vi "Log_ADAM_scan_table.vi"() -> ()   [LabVIEW 2013]
uses:
  ADAM Client/Sub VIs/ADAM Controls/Channel_State.ctl
  Anemometry/Anemometry Sub Vis/Globals/Constants_global.vi
  Anemometry/Anemometry Sub Vis/Globals/Preference_global.vi
  ADAM_Global.vi
  Anemometry/Anemometry Sub Vis/Globals/Meas_global.vi
panel:
  in  "Ventilate Lab if temp above":dbl=21.5
  in  "Averaging time (Seconds)":dbl=60.0
  out "Current time":string
  out "Started Time":string
  in  "stop":bool
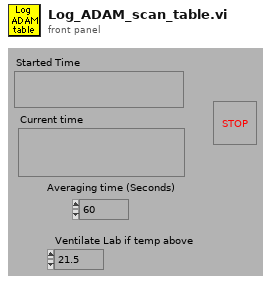
[diagram p1: front panel]
types:
  T1 = enum16{"On", "Off", "Always On", "Always Off", "Delete"}
  T2 = typedef "Channel_State.ctl" = enum16{"On", "Off", "Always On", "Always Off"}
  T3 = enum16{"Load ADAM setup from excel file", "Save ADAM setup to excel file"}
  T4 = cluster{"second":i32, "minute":i32, "hour":i32, "day of month":i32, "month":i32, "year":i32, "day of week":i32, "day of year":i32, "is DST":i32}
  T5 = typedef "Client_State_Cluster.ctl" = cluster{"Client Name":string, "Traverse level State":T6, "People to Email":string[], "Next Contact Time":dbl}
  T6 = typedef "Traverse_Level_State.ctl" = enum16{"Running", "Complete"}
  T7 = typedef "Server_Control.ctl" = cluster{"Channel Name to control":string, "Channel sharing":enum16{"Channel Unshared", "Channel Shared by Rig", "Channel Shared by Group"}, "Default Value":dbl, "Client Array":string[], "Time Stamp":timestamp, "Do Not Reset":bool}
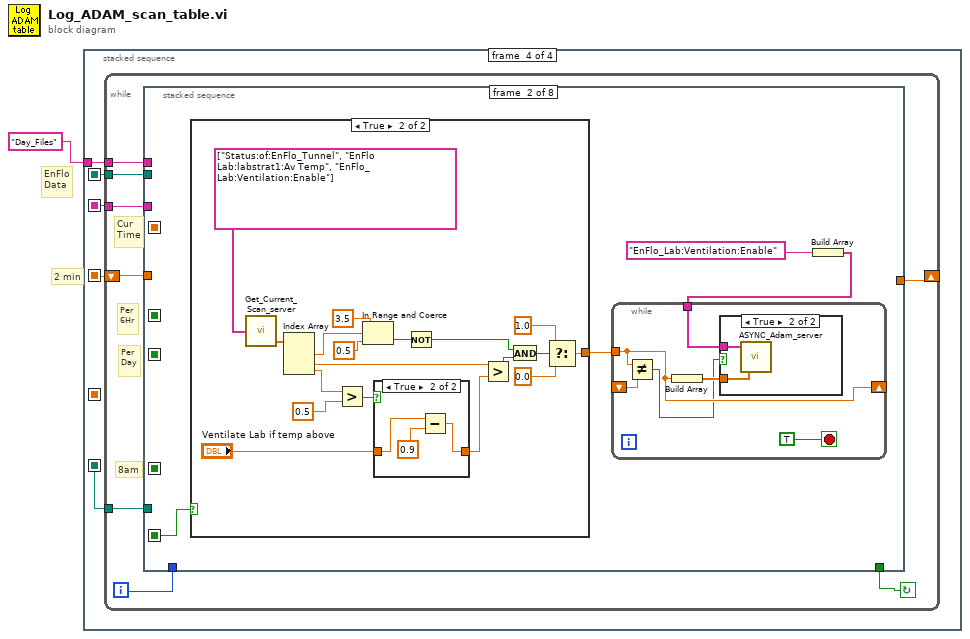
[diagram p0: block diagram]
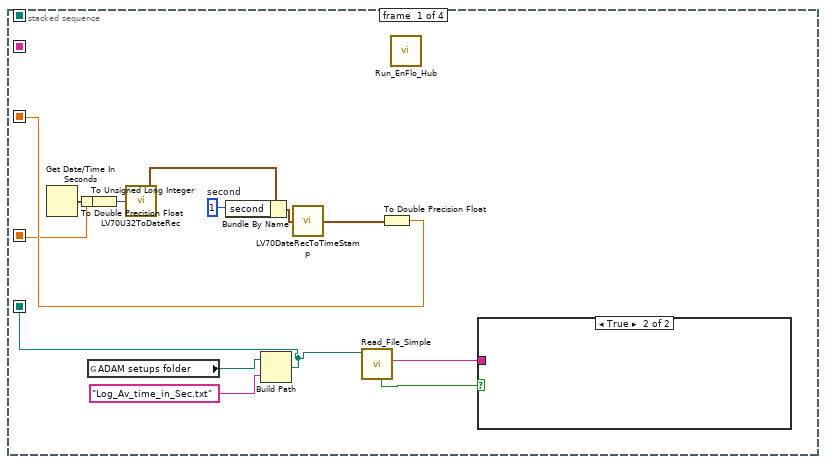
[diagram p2: hidden frame]
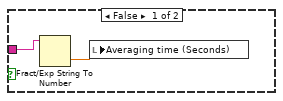
[diagram p3: hidden frame]
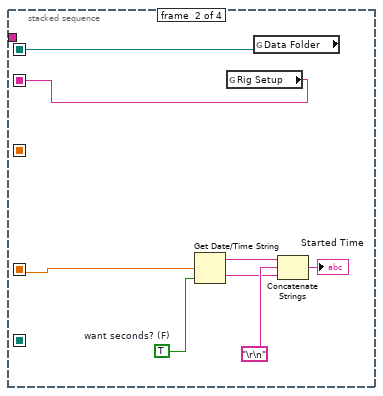
[diagram p4: hidden frame]
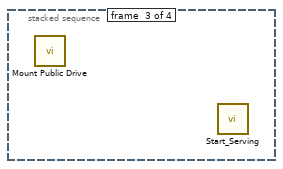
[diagram p5: hidden frame]
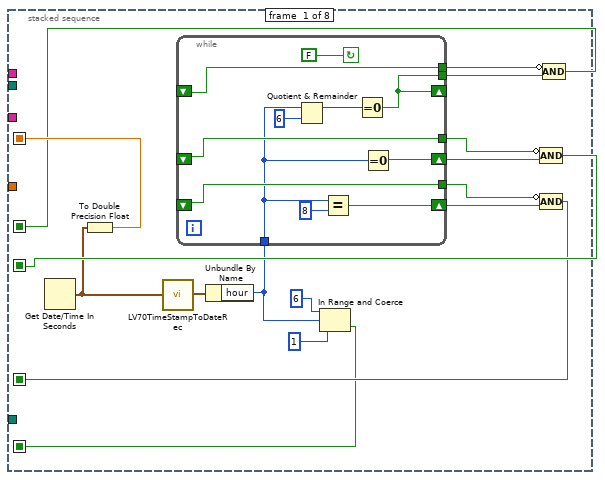
[diagram p6: hidden frame]
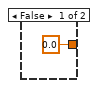
[diagram p8: hidden frame]
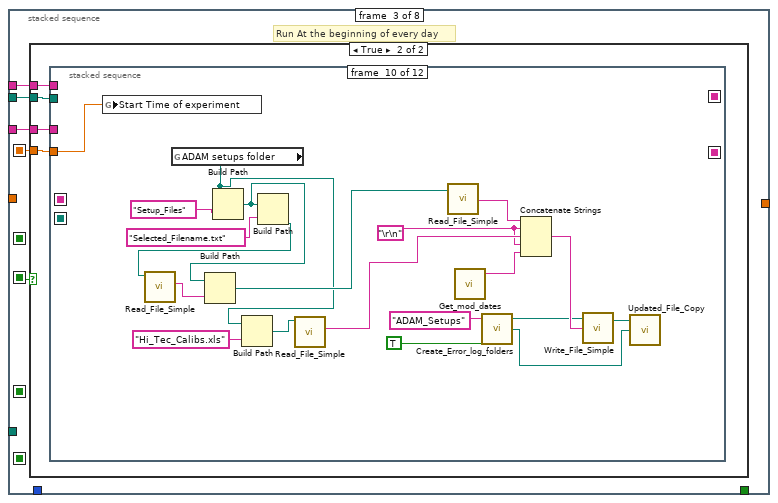
[diagram p10: hidden frame]
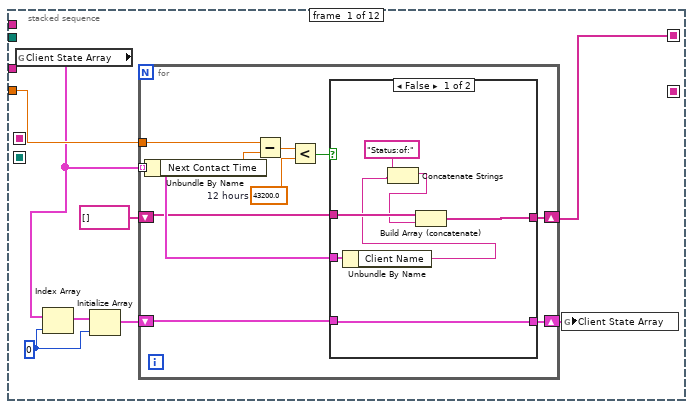
[diagram p12: hidden frame]
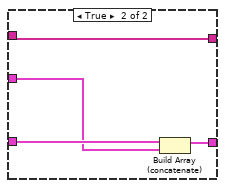
[diagram p13: hidden frame]
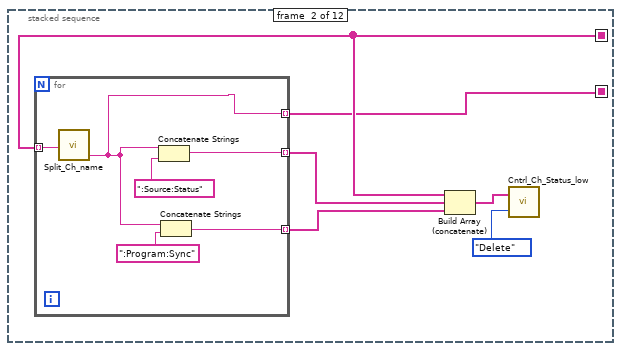
[diagram p14: hidden frame]
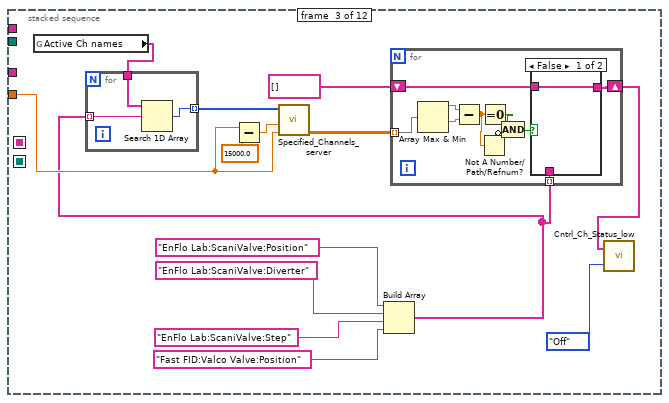
[diagram p15: hidden frame]
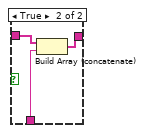
[diagram p16: hidden frame]
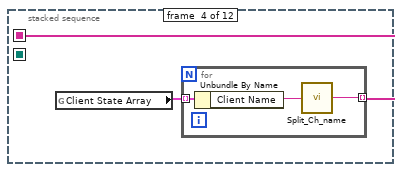
[diagram p17: hidden frame]
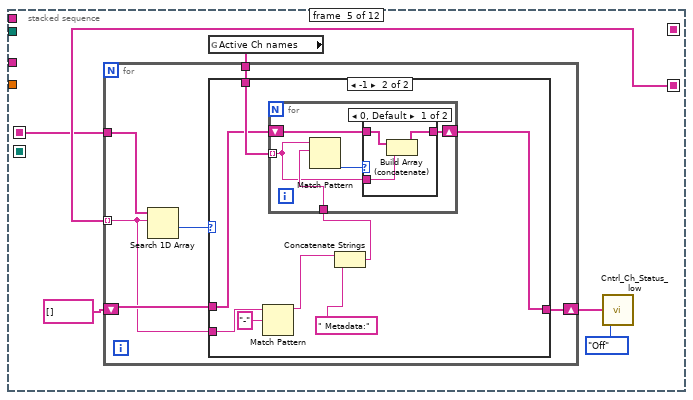
[diagram p18: hidden frame]
diagram:
  # "EnFlo\nData"
  # "2 min"
  n1 = stacked-sequence {
    seq-local: [w12 _ _ _] -> [_ _ _ w29]
    seq-local: [w11 _ _ _] -> [_ w24 _ _]
    seq-local: [_ w18 _ _] -> [_ _ _ w28]
    seq-local: [w4 _ _ _] -> [_ _ _ w26]
    seq-local: [_ w17 _ _] -> [_ _ _ w25]
    tunnel: "Day_Files" ("Input Element") -> [_ _ _ w27]
    frame #0 {
      w14 = 1  # second
      n2 = Get Date/Time In Seconds() -> (seconds since 1Jan1904=w8:timestamp)
      n3 = To Double Precision Float(number=w8) -> (double precision float=w11:dbl)
      n4 = global read "Constants_global.vi" "ADAM setups folder"() -> (w6:path)
      n5 = To Unsigned Long Integer(number=w11) -> (unsigned 32bit integer=w10:u32)
      n6 = call <vilib>:"LV70U32ToDateRec.vi"("Time"=w10) -> ("date time rec"=w9:T4)
      n7 = Bundle By Name(cluster=w9, "second"=w14) -> (w13:T4)
      n8 = Build Path(base path=w6, name or relative path="Log_Av_time_in_Sec.txt") -> (appended path=w4:path)
      n9 = call <vilib>:"LV70DateRecToTimeStamp.vi"("date time rec"=w13) -> ("Time Stamp"=w7:timestamp)
      n10 = call "Read_File_Simple.vi"("Filename"=w4) -> ("Error?"=w2:bool, "string"=w3:string)  [unwired: 2 in, 6 out]
      n11 = To Double Precision Float(number=w7) -> (double precision float=w12:dbl)
      n12 = call "Run_EnFlo_Hub.vi"() -> ()  [unwired: 8 out]
      n13 = case shown="True" w2 {
        tunnel: w3 -> [w16 _]
        frame False {
          n14 = Fract/Exp String To Number(string=w16) -> (number=w15:dbl)  [unwired: 4 out]
          n15 = local write "Averaging time (Seconds)"(w15) -> ()
        }
        frame True {
        }
      }
    }
    frame #1 {
      w23 = TRUE  # want seconds? (F)
      n16 = Get Date/Time String(seconds (now)=w24, want seconds? (F)=w23) -> (date string=w21:string, time string=w20:string)  [unwired: 1 out]
      n17 = global read "Preference_global.vi" "Rig Setup"() -> (w17:string)
      n18 = global read "Constants_global.vi" "Data Folder"() -> (w18:path)
      n19 = Concatenate Strings(w21, "\r\n", w20) -> (→"Started Time":string)
    }
    frame #2 {
      n20 = call "Mount Public Drive.vi"() -> ()  [unwired: 12 in]
      n21 = call "Start_Serving.vi"() -> ()  [unwired: 1 out]
    }
    frame #3 {
      n22 = while {
        tunnel: w28 -> [w35]
        shift-left: w29 -> [w37]
        shift-right: [w36] -> _
        tunnel: w27 -> [w32]
        tunnel: w26 -> [w31]
        tunnel: w25 -> [w30]
        i -> [w34]
        stop <- w33 continue-if-true
        # "8am"
        # "Per\n6Hr"
        # "Per\nDay"
        # "Cur\nTime"
        n23 = stacked-sequence {
          seq-local: [w46 _ _ _ _ _ _ _] -> [_ _ w104 _ _ _ _ _]
          seq-local: [w52 _ _ _ _ _ _ _] -> [_ _ w103 w330 w349 _ _ _]
          seq-local: [w49 _ _ _ _ _ _ _] -> [_ _ _ _ _ _ _ _]
          seq-local: [w42 _ _ _ _ _ _ _] -> [_ _ _ w326 _ _ _ _]
          seq-local: [w38 _ _ _ _ _ _ _] -> [_ w68 _ _ _ _ _ _]
          tunnel: [_ _ _ _ _ w351 _ _] -> w36
          tunnel: w37 -> [_ _ _ _ _ w352 _ _]
          tunnel: w35 -> [_ _ w102 w329 _ w359 _ _]
          tunnel: w34 -> [_ _ _ _ _ _ _ _]
          tunnel: [_ _ _ _ _ _ _ w391] -> w33
          tunnel: w32 -> [_ _ w101 w328 _ w360 _ _]
          tunnel: w31 -> [_ _ _ _ _ _ _ w390]
          tunnel: w30 -> [_ _ w100 w327 _ w353 _ _]
          frame #0 {
            n24 = Get Date/Time In Seconds() -> (seconds since 1Jan1904=w45:timestamp)
            n25 = To Double Precision Float(number=w45) -> (double precision float=w52:dbl)
            n26 = call <vilib>:"LV70TimeStampToDateRec.vi"("time stamp"=w45) -> ("date time rec"=w53:T4)
            n27 = Unbundle By Name(w53) -> ("hour"=w41:i32)
            n28 = while {
              tunnel: [w59] -> w47
              shift-left: _ -> [w59]
              shift-right: [w60] -> w48
              tunnel: [w61] -> w50
              tunnel: [w62] -> w51
              tunnel: w41 -> [w56]
              shift-left: _ -> [w61]
              shift-right: [w62] -> _
              tunnel: [w57] -> w44
              shift-right: [w54] -> w43
              shift-left: _ -> [w57]
              stop <- FALSE continue-if-true
              n29 = Quotient & Remainder(x=w56, y=6) -> (x-y*floor(x/y)=w63:i32)  [unwired: 1 out]
              n30 = Equal?(x=w56, y=8) -> (x = y?=w54:bool)
              n31 = Equal To 0?(x=w63) -> (x = 0?=w62:bool)
              n32 = Equal To 0?(x=w56) -> (x = 0?=w60:bool)
            }
            n33 = In Range and Coerce(upper limit=6, x=w41, lower limit=1) -> (In Range?=w38:bool)  [unwired: 1 out]
            n34 = Compound Arithmetic op=AND(invert w47, w48) -> (w46:bool)
            n35 = Compound Arithmetic op=AND(invert w44, w43) -> (w42:bool)
            n36 = Compound Arithmetic op=AND(invert w50, w51) -> (w49:bool)
          }
          frame #1 {
            n37 = case shown="True" w68 {
              tunnel: [0.0 ("f") w88] -> w65
              frame False {
              }
              frame True {
                n38 = call "Get_Current_Scan_server.vi"("Desired Channels"=string[] ["Status:of:EnFlo_Tunnel", "EnFlo Lab:labstrat1:Av Temp", "EnFlo_Lab:Ventilation:Enable"]) -> ("Numerical Values"=w94:dbl[])  [unwired: 2 out]
                n39 = Index Array(array=w94) -> (element #1=w87:dbl, element #2=w93:dbl, element #3=w82:dbl)  [unwired: 3 in]
                n40 = Greater?(x=w82, y=0.5) -> (0:w80:bool)
                n41 = In Range and Coerce(upper limit=3.5, x=w87, lower limit=0.5) -> (In Range?=w84:bool)  [unwired: 1 out]
                n42 = case shown="True" w80 {
                  tunnel: [w96 w97] -> w79
                  tunnel: "Ventilate Lab if temp above" -> [w96 w99]
                  frame False {
                  }
                  frame True {
                    n43 = Subtract(x=w99, y=0.9) -> (x-y=w97:dbl)
                  }
                }
                n44 = Not(x=w84) -> (.not. x?=w83:bool)
                n45 = Greater?(x=w93, y=w79) -> (0:w92:bool)
                n46 = And(x=w83, y=w92) -> (x .and. y?=w91:bool)
                n47 = Select(t=1.0, s=w91, f=0.0) -> (s? t:f=w88:dbl)
              }
            }
            n48 = Build Array("EnFlo_Lab:Ventilation:Enable") -> (w66:string[])
            n49 = while {
              shift-right: [w72] -> _
              shift-left: _ -> [w73]
              tunnel: w65 -> [w72]
              tunnel: w66 -> [w70]
              stop <- TRUE stop-if-true
              n50 = Not Equal?(x=w72, y=w73) -> (x != y?=w69:bool)
              n51 = Build Array(w72) -> (w74:dbl[])
              n52 = case shown="True" w69 {
                tunnel: w74 -> [_ w76]
                tunnel: w70 -> [_ w75]
                frame False {
                }
                frame True {
                  n53 = call "ASYNC_Adam_server.vi"("Values"=w76, "Channel Names"=w75) -> ()  [unwired: 1 in, 3 out]
                }
              }
            }
          }
          frame #2 {
            # "Run At the beginning of every day"
            n54 = case shown="True" w104 {
              tunnel: w103 -> [_ w108]
              tunnel: w102 -> [_ w107]
              tunnel: w101 -> [_ w106]
              tunnel: w100 -> [_ w105]
              frame False {
              }
              frame True {
                n55 = stacked-sequence {
                  seq-local: [w109 _ _ _ _ _ _ _ _ _ _ _] -> [_ w143 _ _ _ _ _ _ w263 _ _ _]
                  seq-local: [_ w139 _ _ _ _ _ _ _ _ _ _] -> [_ _ _ _ w191 _ _ _ _ _ _ _]
                  seq-local: [_ _ _ w181 _ _ _ _ _ _ _ _] -> [_ _ _ _ w188 _ _ _ _ _ _ _]
                  seq-local: [_ _ _ _ _ _ _ _ _ _ w312 _] -> [_ _ _ _ _ _ _ _ _ _ _ w316]
                  tunnel: w108 -> [w116 _ w160 _ _ _ _ _ _ w310 _ w317]
                  tunnel: w107 -> [_ _ _ _ _ _ _ _ _ _ _ _]
                  tunnel: w106 -> [_ _ _ _ _ _ _ _ _ _ _ _]
                  tunnel: w105 -> [_ _ _ _ _ _ _ _ _ _ _ _]
                  frame #0 {
                    w114 = 0 ("Index")
                    n56 = global read "ADAM_Global.vi" "Client State Array"() -> (w115:T5[])
                    n57 = Index Array(array=w115, index=w114) -> (element=w113:T5)
                    n58 = Initialize Array(w113, w114) -> (w112:T5[])
                    n59 = for {
                      tunnel: w115 -> [w119] mode=indexing
                      shift-right: [w120] -> w111
                      shift-left: w112 -> [w121]
                      tunnel: w116 -> [w126]
                      shift-right: [w117] -> w109
                      shift-left: string[] [] -> [w118]
                      w123 = 43200.0  # 12 hours
                      n60 = Unbundle By Name(w119) -> ("Next Contact Time"=w125:dbl)
                      n61 = Subtract(x=w126, y=w125) -> (x-y=w124:dbl)
                      n62 = Less?(x=w124, y=w123) -> (x < y?=w122:bool)
                      n63 = case shown="False" w122 {
                        tunnel: w121 -> [w133 w137]
                        tunnel: [w133 w136] -> w120
                        tunnel: w119 -> [w132 w135]
                        tunnel: w118 -> [w131 w134]
                        tunnel: [w130 w134] -> w117
                        frame False {
                          n64 = Unbundle By Name(w132) -> ("Client Name"=w128:string)
                          n65 = Concatenate Strings("Status:of:", w128) -> (w127:string)
                          n66 = Build Array (concatenate)(w131, w127) -> (w130:string[])
                        }
                        frame True {
                          n67 = Build Array (concatenate)(w137, w135) -> (w136:T5[])
                        }
                      }
                    }
                    n68 = global write "ADAM_Global.vi" "Client State Array"(w111) -> ()
                  }
                  frame #1 {
                    n69 = for {
                      tunnel: w143 -> [w149] mode=indexing
                      tunnel: [w146] -> w141 mode=indexing
                      tunnel: [w145] -> w140 mode=indexing
                      tunnel: [w144] -> w139 mode=indexing
                      n70 = call "Split_Ch_name.vi"("Ch name"=w149) -> ("Low level"=w144:string)  [unwired: 2 out]
                      n71 = Concatenate Strings(w144, ":Source:Status") -> (w146:string)
                      n72 = Concatenate Strings(w144, ":Program:Sync") -> (w145:string)
                    }
                    n73 = Build Array (concatenate)(w143, w141, w140) -> (w142:string[])
                    n74 = call "Cntrl_Ch_Status_low.vi"("Mode"=T1."Delete", "Channel names"=w142) -> ()  [unwired: 1 out]
                  }
                  frame #2 {
                    n75 = global read "ADAM_Global.vi" "Active Ch names"() -> (w163:string[])
                    n76 = Subtract(x=w160, y=15000.0) -> (x-y=w158:dbl)
                    n77 = Build Array("EnFlo Lab:ScaniValve:Position", "EnFlo Lab:ScaniValve:Diverter", "EnFlo Lab:ScaniValve:Step", "Fast FID:Valco Valve:Position") -> (w156:string[])
                    n78 = for {
                      tunnel: w163 -> [w180]
                      tunnel: w156 -> [w179] mode=indexing
                      tunnel: [w178] -> w161 mode=indexing
                      n79 = Search 1D Array(1D array=w180, element=w179) -> (index of element=w178:i32)  [unwired: 1 out]
                    }
                    n80 = call "Specified_Channels_server.vi"("End time"=w160, "Start time"=w158, "Requested channels"=w161) -> ("Output array"=w157:dbl[][])  [unwired: 2 in, 4 out]
                    n81 = for {
                      tunnel: w157 -> [w170] mode=indexing
                      shift-right: [w171] -> w151
                      shift-left: string[] [] -> [w165]
                      tunnel: w156 -> [w166] mode=indexing
                      n82 = Array Max & Min(array=w170) -> (max value=w173:dbl, min value=w172:dbl)  [unwired: 2 out]
                      n83 = Subtract(x=w173, y=w172) -> (x-y=w169:dbl)
                      n84 = Not A Number/Path/Refnum?(number/path/refnum=w169) -> (NaN/Path/Refnum?=w167:bool)
                      n85 = Equal To 0?(x=w169) -> (x = 0?=w164:bool)
                      n86 = Compound Arithmetic op=AND(w164, invert w167) -> (w168:bool)
                      n87 = case shown="False" w168 {
                        tunnel: [w174 w177] -> w171
                        tunnel: w166 -> [_ w176]
                        tunnel: w165 -> [w174 w175]
                        frame False {
                        }
                        frame True {
                          n88 = Build Array (concatenate)(w175, w176) -> (w177:string[])
                        }
                      }
                    }
                    n89 = call "Cntrl_Ch_Status_low.vi"("Mode"=T1."Off", "Channel names"=w151) -> ()  [unwired: 1 out]
                  }
                  frame #3 {
                    n90 = global read "ADAM_Global.vi" "Client State Array"() -> (w182:T5[])
                    n91 = for {
                      tunnel: w182 -> [w185] mode=indexing
                      tunnel: [w183] -> w181 mode=indexing
                      n92 = Unbundle By Name(w185) -> ("Client Name"=w184:string)
                      n93 = call "Split_Ch_name.vi"("Ch name"=w184) -> ("Middle"=w183:string)  [unwired: 2 out]
                    }
                  }
                  frame #4 {
                    n94 = global read "ADAM_Global.vi" "Active Ch names"() -> (w189:string[])
                    n95 = for {
                      tunnel: w191 -> [w192] mode=indexing
                      shift-right: [w195] -> w187
                      shift-left: string[] [] -> [w196]
                      tunnel: w189 -> [w194]
                      tunnel: w188 -> [w193]
                      n96 = Search 1D Array(1D array=w193, element=w192) -> (index of element=w197:i32)  [unwired: 1 out]
                      n97 = case shown="-1" w197 {
                        tunnel: w196 -> [w198 w204]
                        tunnel: [w198 w203] -> w195
                        tunnel: w192 -> [_ w199]
                        tunnel: w194 -> [_ w205]
                        frame 0, Default {
                        }
                        frame -1 {
                          n98 = Match Pattern(string=w199, regular expression="-") -> (before substring=w200:string)  [unwired: 4 out]
                          n99 = Concatenate Strings(w200, " Metadata:" ("Substring")) -> (w202:string)
                          n100 = for {
                            shift-right: [w209] -> w203
                            shift-left: w204 -> [w210]
                            tunnel: w202 -> [w208]
                            tunnel: w205 -> [w207] mode=indexing
                            n101 = Match Pattern(string=w207, regular expression=w208) -> (offset past match=w211:i32)  [unwired: 4 out]
                            n102 = case shown="0, Default" w211 {
                              tunnel: w210 -> [w213 w215]
                              tunnel: [w212 w215] -> w209
                              tunnel: w207 -> [w214 _]
                              frame 0, Default {
                                n103 = Build Array (concatenate)(w213, w214) -> (w212:string[])
                              }
                              frame -1 {
                              }
                            }
                          }
                        }
                      }
                    }
                    n104 = call "Cntrl_Ch_Status_low.vi"("Mode"=T1."Off", "Channel names"=w187) -> ()  [unwired: 1 out]
                  }
                  frame #5 {
                    n105 = Build Array("EnFlo_Tunnel:Heater:Enable") -> (w221:string[])
                    n106 = call "Get_Current_Scan_server.vi"("Desired Channels"=w221) -> ("Numerical Values"=w220:dbl[])  [unwired: 2 out]
                    n107 = Index Array(array=w220, index=0) -> (element=w218:dbl)
                    n108 = Less?(x=w218, y=0.5) -> (x < y?=w216:bool)
                    n109 = case shown="True" w216 {
                      frame False {
                      }
                      frame True {
                        w227 = "EnFlo_Tunnel:Setpo"
                        n110 = global read "ADAM_Global.vi" "Active Ch names"() -> (w225:string[])
                        n111 = String Length(string=w227) -> (length=w226:i32)
                        n112 = for {
                          shift-right: [w235] -> w224
                          shift-left: string[] [] -> [w237]
                          tunnel: w225 -> [w236] mode=indexing
                          tunnel: w226 -> [w239]
                          tunnel: w227 -> [w238]
                          tunnel: "EnFlo_Tunnel:Power" -> [w233]
                          n113 = String Subset(string=w236, length (rest)=w239) -> (substring=w234:string)  [unwired: 1 out]
                          n114 = Equal?(x=w234, y=w238) -> (x = y?=w231:bool)
                          n115 = Equal?(x=w234, y=w233) -> (x = y?=w232:bool)
                          n116 = Or(x=w231, y=w232) -> (x .or. y?=w230:bool)
                          n117 = case shown="True" w230 {
                            tunnel: w237 -> [w240 w243]
                            tunnel: w236 -> [_ w242]
                            tunnel: [w240 w241] -> w235
                            frame False {
                            }
                            frame True {
                              n118 = Build Array (concatenate)(w243, w242) -> (w241:string[])
                            }
                          }
                        }
                        n119 = call "Adam_Ch_on_off.vi"("Ch State"=Channel_State."Off", "ADAM Ch Names"=w224) -> ()  [unwired: 1 out]
                      }
                    }
                  }
                  frame #6 {
                    n120 = call "Read_Write_ADAM_setup.vi"("Mode"=T3."Save ADAM setup to excel file") -> ()  [unwired: 4 out]
                  }
                  frame #7 {
                    w248 = 5400.0  # 1.5 Hrs in seconds
                    n121 = Build Array("GMU:Source:Meas Q", "GMU:Source:Est Time") -> (w255:string[])
                    n122 = call "Get_Current_Scan_server.vi"("Desired Channels"=w255) -> ("Numerical Values"=w250:dbl[])  [unwired: 2 out]
                    n123 = Index Array(array=w250, index=0 ("Index")) -> (element=w252:dbl)
                    n124 = Index Array(array=w250, index=1 ("Index")) -> (element=w249:dbl)
                    n125 = Less?(x=w252, y=0.01) -> (x < y?=w246:bool)
                    n126 = Greater?(x=w249, y=w248) -> (0:w247:bool)
                    n127 = And(x=w246, y=w247) -> (x .and. y?=w245:bool)
                    n128 = case shown="True" w245 {
                      frame False {
                      }
                      frame True {
                        w258 = FALSE  # Activate channels
                        w259 = enum16{"Channel Name", "Main Address"}."Channel Name" ("Control on")
                        n129 = call "Ch_Active_Control.vi"("Match"="GMU:", "Activate Channels?"=w258, "Control on"=w259) -> ()  [unwired: 1 in, 2 out]
                        n130 = call "Ch_Active_Control.vi"("Match"="source", "Activate Channels?"=w258, "Control on"=w259) -> ()  [unwired: 1 in, 2 out]
                      }
                    }
                  }
                  frame #8 {
                    w267 = 0 ("Index")
                    n131 = global read "ADAM_Global.vi" "Server Control Array"() -> (w264:T7[])
                    n132 = Index Array(array=w264, index=w267) -> (element=w266:T7)
                    n133 = Initialize Array(w266, w267) -> (w265:T7[])
                    n134 = for {
                      tunnel: w264 -> [w269] mode=indexing
                      shift-right: [w274] -> w262
                      shift-left: w265 -> [w275]
                      tunnel: w263 -> [w273]
                      n135 = Unbundle By Name(w269) -> ("Client Array"=w272:string[])
                      n136 = for {
                        tunnel: w273 -> [w280]
                        tunnel: w272 -> [w278] mode=indexing
                        shift-right: [w276] -> w268
                        shift-left: string[] [] -> [w277]
                        n137 = Search 1D Array(1D array=w280, element=w278) -> (index of element=w279:i32)  [unwired: 1 out]
                        n138 = case shown="0, Default" w279 {
                          tunnel: w278 -> [_ w284]
                          tunnel: w277 -> [w281 w283]
                          tunnel: [w281 w282] -> w276
                          frame 0, Default {
                          }
                          frame -1 {
                            n139 = Build Array (concatenate)(w283, w284) -> (w282:string[])
                          }
                        }
                      }
                      n140 = Array Size(array=w268) -> (size(s)=w270:i32)
                      n141 = case shown="0" w270 {
                        tunnel: w275 -> [w285 w289]
                        tunnel: [w285 w290] -> w274
                        tunnel: w269 -> [_ w288]
                        tunnel: w268 -> [_ w287]
                        frame 0 {
                        }
                        frame 1, Default {
                          n142 = Bundle By Name(cluster=w288, "Client Array"=w287) -> (w286:T7)
                          n143 = Build Array (concatenate)(w289, w286) -> (w290:T7[])
                        }
                      }
                    }
                    n144 = global write "ADAM_Global.vi" "Server Control Array"(w262) -> ()
                  }
                  frame #9 {
                    w298 = "\r\n"
                    n145 = global write "Meas_global.vi" "Start Time of experiment"(w310) -> ()
                    n146 = global read "Constants_global.vi" "ADAM setups folder"() -> (w301:path)
                    n147 = Build Path(base path=w301, name or relative path="Setup_Files") -> (appended path=w305:path)
                    n148 = Build Path(base path=w301, name or relative path="Hi_Tec_Calibs.xls") -> (appended path=w300:path)
                    n149 = Build Path(base path=w305, name or relative path="Selected_Filename.txt" ("Substring")) -> (appended path=w307:path)
                    n150 = call "Read_File_Simple.vi"("Filename"=w307) -> ("string"=w306:string)  [unwired: 2 in, 7 out]
                    n151 = Build Path(base path=w305, name or relative path=w306) -> (appended path=w304:path)
                    n152 = call "Read_File_Simple.vi"("Filename"=w300) -> ("string"=w299:string)  [unwired: 2 in, 7 out]
                    n153 = call "Read_File_Simple.vi"("Filename"=w304) -> ("string"=w303:string)  [unwired: 2 in, 7 out]
                    n154 = call "Get_mod_dates.vi"() -> ("Output string"=w297:string)  [unwired: 1 in, 4 out]
                    n155 = call "Create_Error_log_folders.vi"("Per Day Log File?"=TRUE, "Log Filename"="ADAM_Setups" ("Substring")) -> ("Server copy Location"=w291:path, "Local Log File"=w293:path)  [unwired: 1 in, 1 out]
                    n156 = Concatenate Strings(w303, w298, w299, w298, w297) -> (w294:string)
                    n157 = call "Write_File_Simple.vi"("character string"=w294, "file path"=w293) -> ("file path Out"=w292:path)  [unwired: 1 in, 1 out]
                    n158 = call "Updated_File_Copy.vi"("Target Path"=w291, "Source Path"=w292) -> ()  [unwired: 2 out]
                  }
                  frame #10 {
                    n159 = global read "Constants_global.vi" "Data Folder Local"() -> (w313:path)
                    n160 = Build Path(base path=w313, name or relative path="Results_Summary_files") -> (appended path=w312:path)
                  }
                  frame #11 {
                    # "If the summary files are more than 60 days old delete them"
                    n161 = To Unsigned Long Integer(number=w317) -> (unsigned 32bit integer=w314:u32)
                    n162 = call "Get_folder_and_filenames.vi"("file path (dialog if empty)"=w316) -> ("Files"=w315:path[])  [unwired: 1 out]
                    n163 = for {
                      tunnel: w315 -> [w319] mode=indexing
                      tunnel: w314 -> [w324]
                      # "60 days in seconds"
                      n164 = File/Directory Info(path=w319) -> (last mod=w318:timestamp)  [unwired: 1 in, 6 out]
                      n165 = To Unsigned Long Integer(number=w318) -> (unsigned 32bit integer=w323:u32)
                      n166 = Subtract(x=w324, y=w323) -> (x-y=w322:u32)
                      n167 = Greater?(x=w322, y=u32 5184000) -> (0:w320:bool)
                      n168 = case shown="False" w320 {
                        tunnel: w319 -> [_ w325]
                        frame False {
                        }
                        frame True {
                          n169 = Delete(path (use dialog)=w325) -> ()  [unwired: 1 in, 6 out]
                        }
                      }
                    }
                  }
                }
              }
            }
          }
          frame #3 {
            # "At 8am every day"
            n170 = case shown="True" w326 {
              tunnel: w330 -> [_ w334]
              tunnel: w329 -> [_ w333]
              tunnel: w328 -> [_ w332]
              tunnel: w327 -> [_ w331]
              frame False {
              }
              frame True {
                n171 = stacked-sequence {
                  seq-local: [w342 _] -> [_ w348]
                  tunnel: w334 -> [w346 _]
                  tunnel: w333 -> [w335 _]
                  tunnel: w332 -> [w340 _]
                  tunnel: w331 -> [w336 _]
                  frame #0 {
                    n172 = Subtract(x=w346, y=36000.0) -> (x-y=w344:dbl)
                    n173 = call "Sec_to_date_filename.vi"("seconds"=w344) -> ("Year"=w341:string, "Month"=w345:string, "Day"=w338:string)  [unwired: 1 out]
                    n174 = Concatenate Strings(w338, ".xls" ("string")) -> (w337:string)
                    n175 = Build Array(w341, w336, w340, w345, w337) -> (w343:string[])
                    n176 = call "Build_Pathname.vi"("PathElements"=w343, "PathnameIn"=w335) -> ("AppendedPath"=w342:path)
                  }
                  frame #1 {
                    # "This VI emails a summary of all the server errors that occured Yesterday"
                    n177 = call "Adam_server_messages.vi"("Filename"=w348) -> ()  [unwired: 1 out]
                  }
                }
              }
            }
          }
          frame #4 {
            n178 = call "EnFlo_Seeder_Control.vi"("Current Time (s)"=w349) -> ()
            n179 = Wait (ms)(milliseconds to wait=u32 1000 ("milliseconds to Wait")) -> ()  [unwired: 1 out]
          }
          frame #5 {
            n180 = Divide(x="Averaging time (Seconds)", y=60.0) -> (x/y=w357:dbl)
            n181 = Divide(x="Averaging time (Seconds)", y=2.0) -> (x/y=w354:dbl)
            n182 = Add(x=w354, y=w352) -> (x+y=w370:dbl)
            n183 = call "Sec_to_date_filename.vi"("seconds"=w370) -> ("Year"=w365:string, "Month"=w366:string, "Day"=w361:string)  [unwired: 1 out]
            n184 = Concatenate Strings(w361, ".xls" ("string")) -> (w363:string)
            n185 = Build Array(w365, w353, w360, w366, w363) -> (w364:string[])
            n186 = call "Time_elapsed.vi"("End of previous average in"=w352, "Averaging time (mins)"=w357) -> ("End of previous average out"=w351:dbl, "End of period"=w368:dbl, "Start of period"=w369:dbl, "Time elapsed ?"=w367:bool)  [unwired: 2 in]
            n187 = case shown="True" w367 {
              tunnel: w368 -> [_ w373]
              tunnel: w369 -> [_ w374]
              tunnel: w359 -> [_ w372]
              tunnel: w364 -> [_ w371]
              frame False {
              }
              frame True {
                n188 = stacked-sequence {
                  tunnel: w374 -> [w383 _]
                  tunnel: w373 -> [w382 _]
                  tunnel: w372 -> [w375 _]
                  tunnel: w371 -> [w378 _]
                  frame #0 {
                    n189 = global read "ADAM_Global.vi" "2 Min average comment"() -> (w381:string)
                    n190 = global read "Meas_global.vi" "Error Messages"() -> (w380:string)
                    n191 = call "Build_Pathname.vi"("PathElements"=w378, "PathnameIn"=w375) -> ("AppendedPath"=w377:path)
                    n192 = call "Create_directory_path.vi"("Path name"=w377) -> ("Path name Out"=w376:path)  [unwired: 1 in, 1 out]
                    n193 = Concatenate Strings(w381, w380) -> (w379:string)
                    n194 = call "Write_to_log_file.vi"("User added comment"=w379, "End time"=w382, "Start time"=w383, "Folder/file"=w376) -> ()  [unwired: 5 in, 3 out]
                  }
                  frame #1 {
                    w384 = ""
                    n195 = global write "ADAM_Global.vi" "2 Min average comment"(w384) -> ()
                    n196 = global write "Meas_global.vi" "Error Messages"(w384) -> ()
                  }
                }
              }
            }
          }
          frame #6 {
            w389 = TRUE  # want seconds? (F)
            n197 = Get Date/Time String(want seconds? (F)=w389) -> (date string=w387:string, time string=w386:string)  [unwired: 2 out]
            n198 = Concatenate Strings(w387, "\r\n", w386) -> (→"Current time":string)
          }
          frame #7 {
            n199 = while {
              shift-right: [w393] -> _
              shift-left: _ -> [w397]
              tunnel: w390 -> [w394]
              stop <- TRUE stop-if-true
              n200 = local read "Averaging time (Seconds)"() -> (w393:dbl)
              n201 = Not Equal?(x=w393, y=w397) -> (x != y?=w395:bool)
              n202 = case shown="True" w395 {
                tunnel: w394 -> [_ w398]
                tunnel: w393 -> [_ w400]
                frame False {
                }
                frame True {
                  n203 = Number To Fractional String(number=w400, precision (6)=i16 6) -> (F-format string=w399:string)  [unwired: 2 out]
                  n204 = call "Write_File_Simple.vi"("character string"=w399, "file path"=w398) -> ()  [unwired: 1 in, 2 out]
                }
              }
            }
            n205 = Not(x="stop") -> (.not. x?=w391:bool)
          }
        }
      }
    }
  }
